vi "Remote PC - Client_DUT2.vi"(6 "Remote Sever Port (2800)":u16, 7 "Flow Contorl":enum16{"Connect", "Read", "Write", "Close"}(ring)=enum."Write", 8 "error in":errorcluster, 9 "Send Command":T1="Analyze Log", 10 "Log Path":path=path "D:/My Projects/MitraStar/wlan test lib - onsite - second round/Report SubVIs/DUT 1_9_09_38 AM 10_24_2013_Report.csv", 11 "IP Address":string="localhost") -> (0 "error out":errorcluster, 1 "Receive Message":string, 3 "MAC&SN":string)   [LabVIEW 2012]
uses:
  TypeDef/Send Command Message.ctl
panel:
  out "bytes written":i32=19538
  out "data out":string="DONE\r\n"
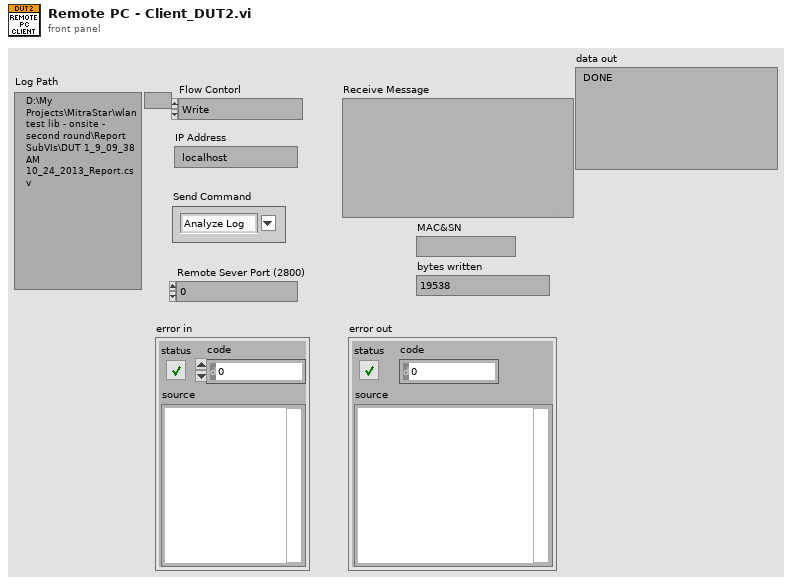
[diagram p1: front panel]
types:
  T1 = typedef "Send Command Message.ctl" = string
  T2 = enum16{"Standard", "Buffered", "CRLF", "Immediate"}
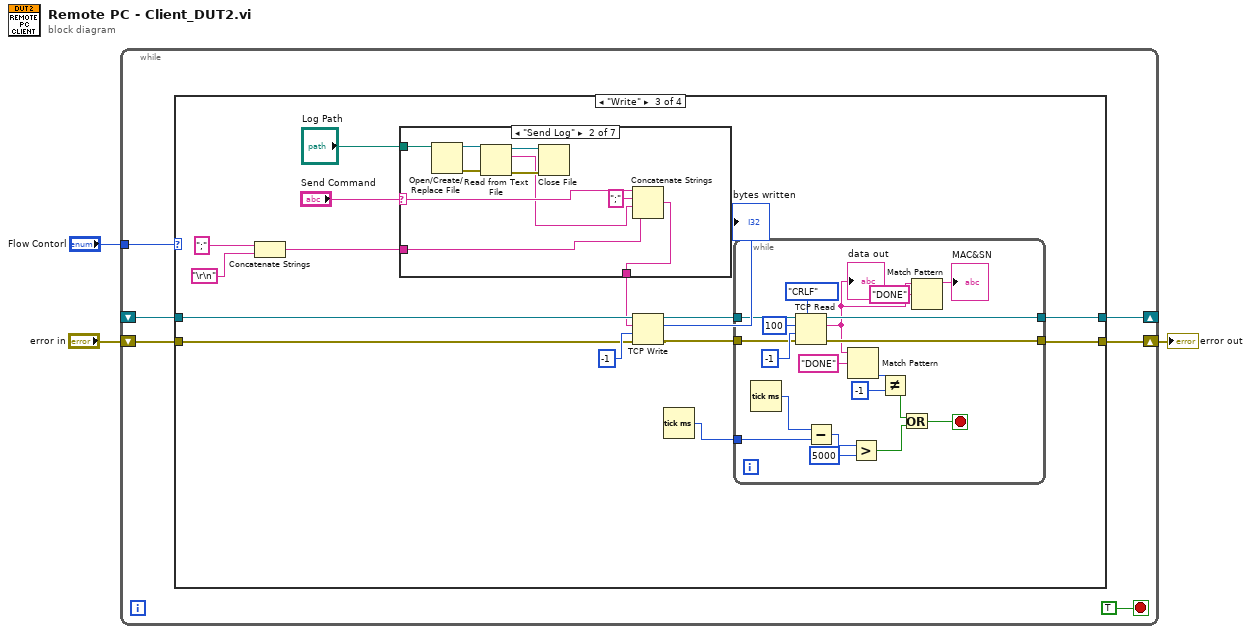
[diagram p0: block diagram]
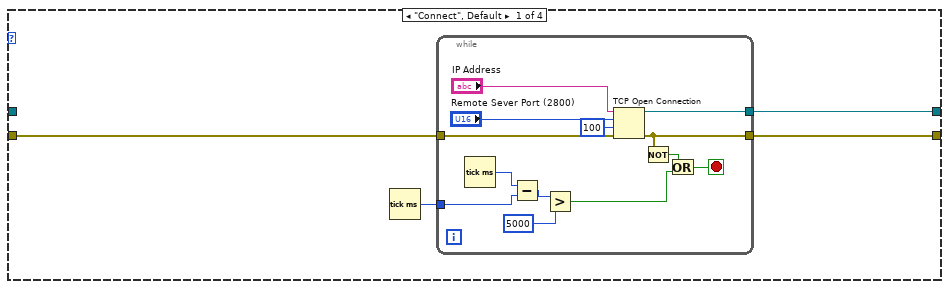
[diagram p2: hidden frame]
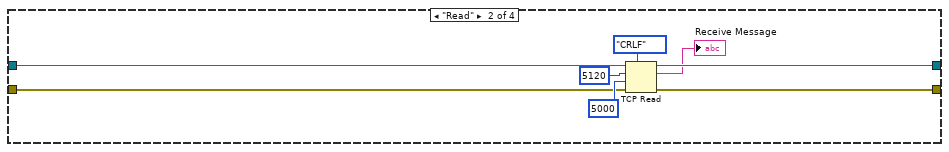
[diagram p3: hidden frame]
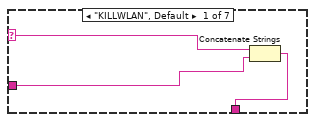
[diagram p4: hidden frame]
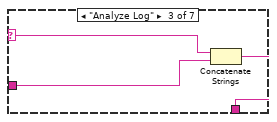
[diagram p5: hidden frame]
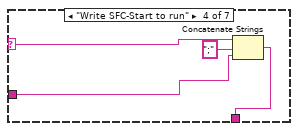
[diagram p6: hidden frame]
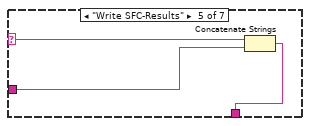
[diagram p7: hidden frame]
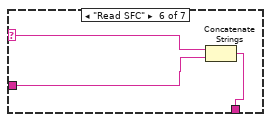
[diagram p8: hidden frame]
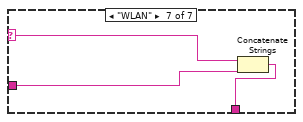
[diagram p9: hidden frame]
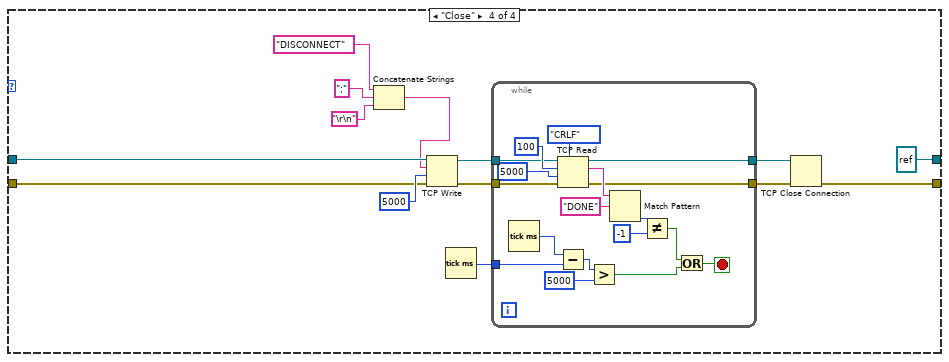
[diagram p10: hidden frame]
diagram:
  n1 = while {
    shift-right: [w7] -> w2
    shift-left: "error in" -> [w8]
    shift-right: [w6] -> _
    shift-left: _ -> [w5]
    tunnel: "Flow Contorl" -> [w4]
    stop <- TRUE stop-if-true
    n2 = case shown="\"Write\"" w4 {
      tunnel: w8 -> [w13 w30 w47 w109]
      tunnel: [w12 w29 w43 w112] -> w7
      tunnel: [w11 w28 w44 refnum<k5> refnum ("connection ID")] -> w6
      tunnel: w5 -> [_ w31 w48 w108]
      frame "Connect", Default {
        n3 = Tick Count (ms)() -> (millisecond timer value=w10:u32)
        n4 = while {
          tunnel: w13 -> [w24]
          tunnel: [w15] -> w12
          tunnel: [w23] -> w11
          tunnel: w10 -> [w20]
          stop <- w16 stop-if-true
          n5 = Tick Count (ms)() -> (millisecond timer value=w21:u32)
          n6 = Subtract(x=w21, y=w20) -> (x-y=w19:u32)
          n7 = Greater?(x=w19, y=u32 5000) -> (0:w17:bool)
          n8 = TCP Open Connection(address="IP Address", remote port or service name="Remote Sever Port (2800)", timeout ms (60000)=100, error in (no error)=w24) -> (connection ID=w23:refnum<k5>, error out=w15:errorcluster)  [unwired: 1 in]
          n9 = Not(x=w15) -> (.not. x?=w14:bool)
          n10 = Or(x=w14, y=w17) -> (x .or. y?=w16:bool)
        }
      }
      frame "Read" {
        n11 = TCP Read(connection ID=w31, bytes to read=5120, error in (no error)=w30, 7:T2."CRLF" ("mode (standard)"), 9:5000 ("timeout ms (25000)")) -> (connection ID out=w28:refnum<k5>, data out=→"Receive Message":string, error out=w29:errorcluster)
      }
      frame "Write" {
        n12 = Concatenate Strings(";", "\r\n") -> (w38:string)
        n13 = case shown="\"Send Log\"" "Send Command" {
          selector: "Send Command" -> [w52 w61 w65 w68 w72 w75 w78]
          tunnel: [w51 w62 w64 w69 w70 w74 w77] -> w41
          tunnel: w38 -> [w50 w59 w63 w66 w71 w73 w76]
          tunnel: "Log Path" -> [_ w53 _ _ _ _ _]
          frame "KILLWLAN", Default {
            n14 = Concatenate Strings(w52, w50) -> (w51:string)
          }
          frame "Send Log" {
            n15 = Open/Create/Replace File(file path (use dialog)=w53) -> (refnum out=w56:refnum<file>, error out=w55:errorcluster)  [unwired: 5 in, 1 out]
            n16 = Read from Text File(file (use dialog)=w56, error in=w55) -> (refnum out=w58:refnum<file>, text=w54:string, error out=w57:errorcluster)  [unwired: 2 in, 1 out]
            n17 = Close File(refnum=w58, error in=w57) -> ()  [unwired: 2 out]
            n18 = Concatenate Strings(w61, ";" ("string"), w54, w59) -> (w62:string)
          }
          frame "Analyze Log" {
            n19 = Concatenate Strings(w65, w63) -> (w64:string)
          }
          frame "Write SFC-Start to run" {
            n20 = Concatenate Strings(w68, ";" ("string"), w66) -> (w69:string)
          }
          frame "Write SFC-Results" {
            n21 = Concatenate Strings(w72, w71) -> (w70:string)
          }
          frame "Read SFC" {
            n22 = Concatenate Strings(w75, w73) -> (w74:string)
          }
          frame "WLAN" {
            n23 = Concatenate Strings(w78, w76) -> (w77:string)
          }
        }
        n24 = TCP Write(connection ID=w48, data in=w41, error in (no error)=w47, 9:-1 ("timeout ms (25000)")) -> (connection ID out=w45:refnum<k5>, bytes written=→"bytes written":i32, error out=w46:errorcluster)
        n25 = Tick Count (ms)() -> (millisecond timer value=w35:u32)
        n26 = while {
          tunnel: [w92] -> w44
          tunnel: [w91] -> w43
          tunnel: w45 -> [w90]
          tunnel: w46 -> [w89]
          tunnel: w35 -> [w84]
          stop <- w79 stop-if-true
          n27 = Tick Count (ms)() -> (millisecond timer value=w85:u32)
          n28 = TCP Read(connection ID=w90, bytes to read=100, error in (no error)=w89, 7:T2."CRLF" ("mode (standard)"), 9:-1 ("timeout ms (25000)")) -> (connection ID out=w92:refnum<k5>, data out=w88:string, error out=w91:errorcluster)
          "data out" <- w88
          n29 = Subtract(x=w85, y=w84) -> (x-y=w83:u32)
          n30 = Match Pattern(string=w88, regular expression="DONE") -> (offset past match=w95:i32)  [unwired: 1 in, 3 out]
          n31 = Greater?(x=w83, y=u32 5000) -> (0:w80:bool)
          n32 = Not Equal?(x=w95, y=-1) -> (x != y?=w81:bool)
          n33 = Or(x=w81, y=w80) -> (x .or. y?=w79:bool)
          n34 = Match Pattern(string=w88, regular expression="DONE") -> (before substring=→"MAC&SN":string)  [unwired: 1 in, 3 out]
        }
      }
      frame "Close" {
        n35 = Concatenate Strings("DISCONNECT" ("data in"), ";", "\r\n") -> (w99:string)
        n36 = TCP Write(connection ID=w108, data in=w99, error in (no error)=w109, 9:5000 ("timeout ms (25000)")) -> (connection ID out=w104:refnum<k5>, error out=w103:errorcluster)  [unwired: 1 out]
        n37 = Tick Count (ms)() -> (millisecond timer value=w107:u32)
        n38 = while {
          tunnel: w107 -> [w122]
          tunnel: [w116] -> w106
          tunnel: [w115] -> w105
          tunnel: w104 -> [w114]
          tunnel: w103 -> [w113]
          stop <- w117 stop-if-true
          n39 = Tick Count (ms)() -> (millisecond timer value=w123:u32)
          n40 = TCP Read(connection ID=w114, bytes to read=100, error in (no error)=w113, 7:T2."CRLF" ("mode (standard)"), 9:5000 ("timeout ms (25000)")) -> (connection ID out=w116:refnum<k5>, data out=w128:string, error out=w115:errorcluster)
          n41 = Subtract(x=w123, y=w122) -> (x-y=w121:u32)
          n42 = Greater?(x=w121, y=u32 5000) -> (0:w118:bool)
          n43 = Match Pattern(string=w128, regular expression="DONE") -> (offset past match=w126:i32)  [unwired: 1 in, 3 out]
          n44 = Not Equal?(x=w126, y=-1) -> (x != y?=w119:bool)
          n45 = Or(x=w119, y=w118) -> (x .or. y?=w117:bool)
        }
        n46 = TCP Close Connection(connection ID=w106, error in (no error)=w105) -> (error out=w112:errorcluster)  [unwired: 1 in, 1 out]
      }
    }
  }
  "error out" <- w2
